vi "Teleop.vi"(10 "Match Info":T1={"Autonomous Elapsed Seconds"=0.0, "TeleOp Elapsed Seconds"=0.0, "Disabled Elapsed Seconds"=0.0, "Visited Autonomous"=FALSE, "Visited TeleOp"=FALSE, "Visited Disabled"=FALSE, "Autonomous Settings"={"Autonomous Style"=enum."Independent", "VI Refnum"=refnum}}, 11 "Call Context":T2) -> ()   [LabVIEW 2019]
doc: "This VI is called for each TeleOp packet received from the DS where the robot is not disabled. It is often used to read from the joysticks and update I/O or to update setpoints for timed control loops. It should complete and return within 20 milliseconds or it may miss DS packets."
uses:
  <vilib>/Rock Robotics/WPI/DriverStation/WPI_DriverStationDerivedRobotMode.ctl
  <vilib>/Rock Robotics/WPI/DriverStation/WPI_DriverStationMatch Info.ctl
  <vilib>/Rock Robotics/WPI/Solenoid/WPI_SolenoidValue.ctl
  <vilib>/Rock Robotics/Network Tables/NT Read Boolean.vi
  <vilib>/Rock Robotics/Network Tables/NT Read Number.vi
  <vilib>/Rock Robotics/WPI/Utilities/WPI_GetSetVariantRefNum.vi
  <vilib>/Rock Robotics/Network Tables/NT Write Boolean Array.vi
  <vilib>/Rock Robotics/Network Tables/NT Write Numeric Array.vi
  <vilib>/Rock Robotics/WPI/RobotDrive/WPI_RobotDriveArcadeDrive_Standard(NoSaturation).vi
  <vilib>/Rock Robotics/WPI/Solenoid/WPI_SolenoidSetEnum.vi
panel:
  out "Sample Slider 0":dbl(slide) scale=0.0..5.0
  out "Sample Boolean 1":bool
  out "Sample Boolean 0":bool
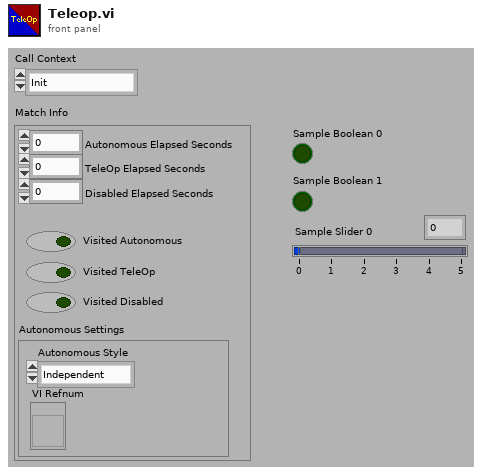
[diagram p1: front panel]
types:
  T1 = typedef "WPI_DriverStationMatch Info.ctl" = cluster{"Autonomous Elapsed Seconds":dbl, "TeleOp Elapsed Seconds":dbl, "Disabled Elapsed Seconds":dbl, "Visited Autonomous":bool, "Visited TeleOp":bool, "Visited Disabled":bool, "Autonomous Settings":cluster{"Autonomous Style":enum16{"Iterative", "Independent"}, "VI Refnum":refnum<vi>}}
  T2 = typedef "WPI_DriverStationDerivedRobotMode.ctl" = enum16{"Init", "Execute", "Stop"}
  T3 = typedef "WPI_JoystickDevRef.ctl" = cluster{"Device":T4}
  T4 = typedef "WPI_JoystickDeviceEnum.ctl" = enum16{"USB 0", "USB 1", "USB 2", "USB 3", "USB 4", "USB 5"}
  T5 = typedef "WPI_MotorControlDeviceRef.ctl" = cluster{"DeviceStatus":errorcluster, "Type":T6, "PWM":cluster{"PWM Channel":T7, "DeadBand":T8}, "CAN":cluster{"Device Number":u8, "SetOutput VI Ref":variant, "GetOutput VI Ref":variant, "Enable VI Ref":variant, "Disable VI Ref":variant, "Data":variant}, "Invert":bool, "DIO PWM":cluster{"PWM \"Enable\" Channel":T7, "DIOChannel":T9, "PWM Rate":dbl}}
  T6 = typedef "WPI_MotorControlType.ctl" = enum16{"PWM", "CAN", "DIO PWM"}
  T7 = typedef "FPGA_DIOPWMChannel.ctl" = enum8{"PWM 0", "PWM 1", "PWM 2", "PWM 3", "PWM 4", "PWM 5", "PWM 6", "PWM 7", "PWM 8", "PWM 9", "PWM MXP 0", "PWM MXP 1", "PWM MXP 2", "PWM MXP 3", "PWM MXP 4", "PWM MXP 5", "PWM MXP 6", "PWM MXP 7", "PWM MXP 8", "PWM MXP 9", "Invalid"}
  T8 = typedef "WPI_PWMDeadband.ctl" = cluster{"Name":string, "maxPositivePwm":i32, "minPositivePwm":i32, "centerPwm":i32, "maxNegativePwm":i32, "minNegativePwm":i32, "angularRange":u16}
  T9 = typedef "FPGA_DIOChannel.ctl" = enum8{"DIO 0", "DIO 1", "DIO 2", "DIO 3", "DIO 4", "DIO 5", "DIO 6", "DIO 7", "DIO 8", "DIO 9", "DIO MXP 0", "DIO MXP 1", "DIO MXP 2", "DIO MXP 3", "DIO MXP 4", "DIO MXP 5", "DIO MXP 6", "DIO MXP 7", "DIO MXP 8", "DIO MXP 9", "DIO MXP 10", "DIO MXP 11", "DIO MXP 12", "DIO MXP 13", "DIO MXP 14", "DIO MXP 15", "SPI Port CS1", "SPI Port CS2", "SPI Port CS3", "SPI Port MISO", "SPI Port MOSI", "Invalid"}
  T10 = typedef "WPI_SolenoidValue.ctl" = enum16{"Off", "On", "Forward", "Reverse"}
  T11 = typedef "WPI_SolenoidDevRef.ctl" = cluster{"DevStatus":errorcluster, "Pneumatics Control Module":u8, "Forward Solenoid Channel":T12, "Reverse Solenoid Channel":T12}
  T12 = typedef "WPI_SolenoidChannel.ctl" = enum8{"Solenoid 0", "Solenoid 1", "Solenoid 2", "Solenoid 3", "Solenoid 4", "Solenoid 5", "Solenoid 6", "Solenoid 7", "Invalid"}
  T13 = typedef "WPI_RobotDriveDevRef.ctl" = cluster{"DevStatus":errorcluster, "Motors[]":T5[], "Square Inputs":bool, "Max Output":dbl}
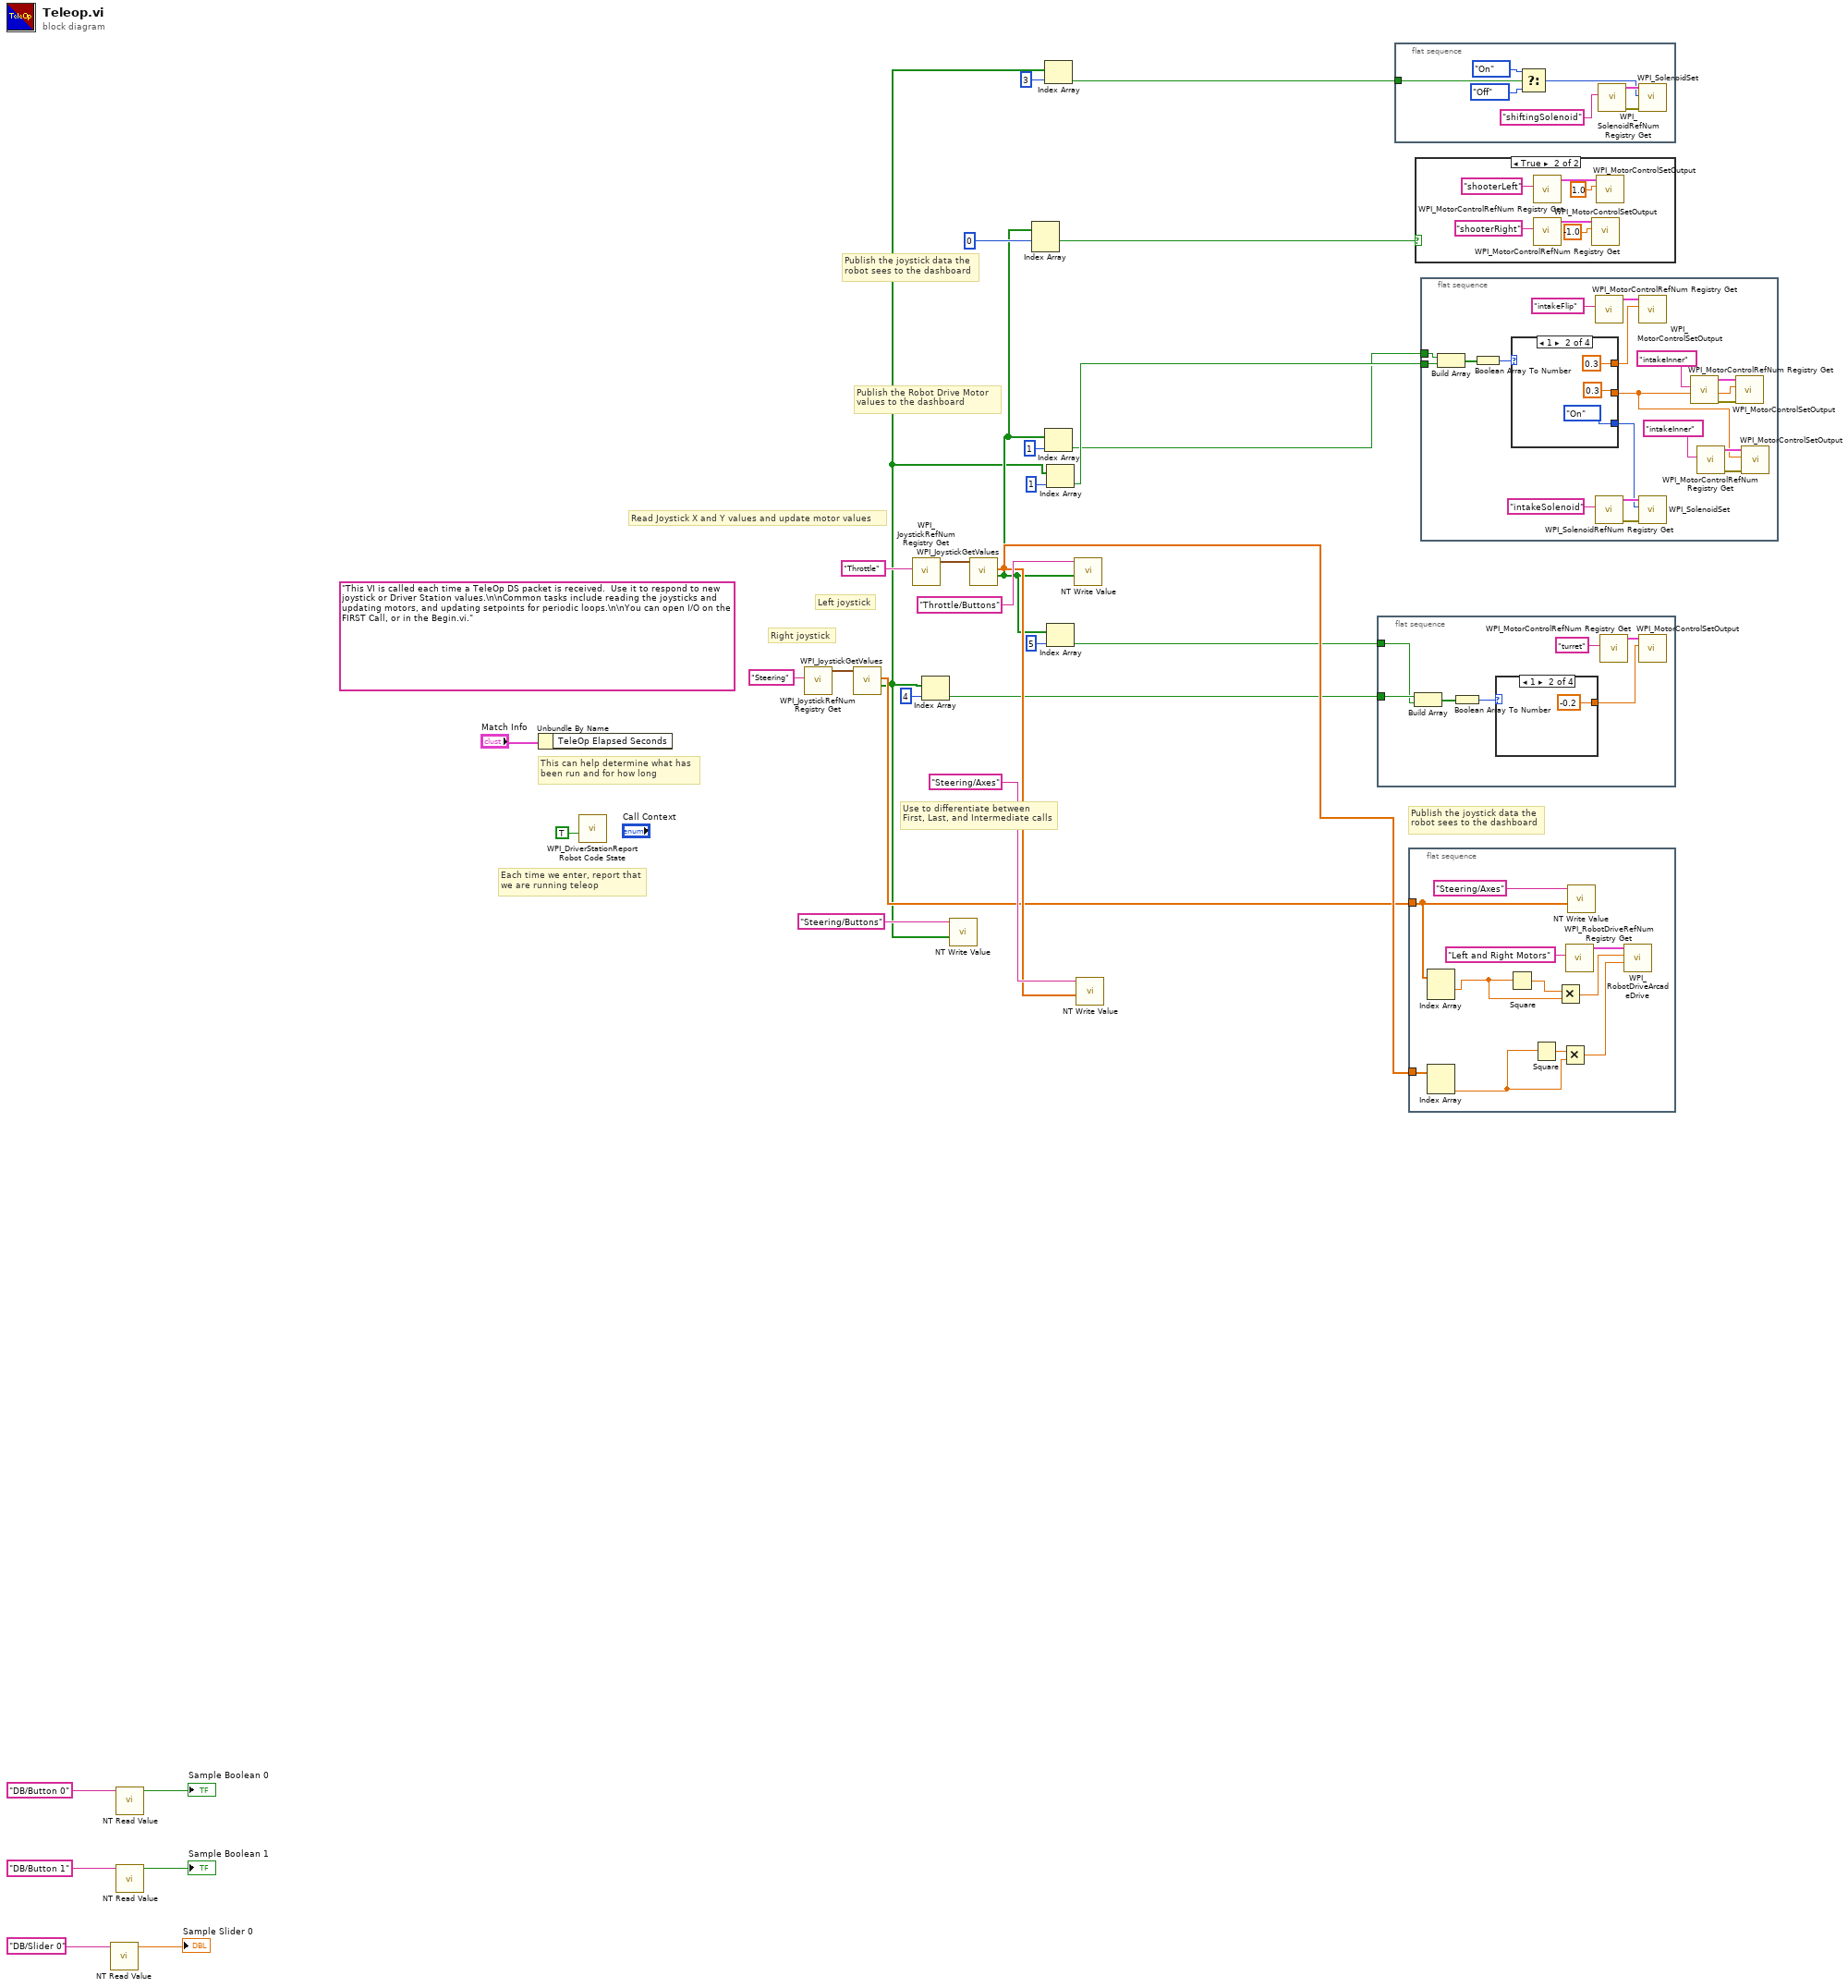
[diagram p0: block diagram]
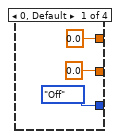
[diagram p2: hidden frame]
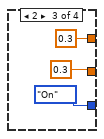
[diagram p3: hidden frame]
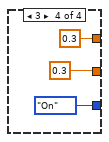
[diagram p4: hidden frame]
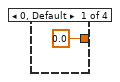
[diagram p5: hidden frame]
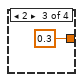
[diagram p6: hidden frame]
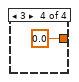
[diagram p7: hidden frame]
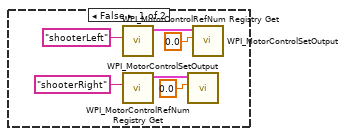
[diagram p8: hidden frame]
diagram:
  (unwired) "This VI is called each time a TeleOp DS packet is received.  Use it to respond to new joystick or Driver Station values.\n\nCommon tasks include reading the joysticks and updating motors, and updating setpoints for periodic loops.\n\nYou can open I/O on the FIRST Call, or in the Begin.vi."
  # "Right joystick"
  # "Left joystick"
  # "Publish the Robot Drive Motor\nvalues to the dashboard"
  # "Publish the joystick data the\nrobot sees to the dashboard"
  # "Publish the joystick data the\nrobot sees to the dashboard"
  # "Each time we enter, report that\nwe are running teleop"
  # "Use to differentiate between\nFirst, Last, and Intermediate calls"
  # "This can help determine what has\nbeen run and for how long"
  # "Read Joystick X and Y values and update motor values"
  n1 = call-poly <vilib>:"NT Read Value.vi"("Name"="DB/Slider 0" ("refnum name")) -> ("Numeric"=→"Sample Slider 0":dbl)  [unwired: 9 in, 1 out]
  n2 = call-poly <vilib>:"NT Read Value.vi"("Name"="DB/Button 0" ("refnum name")) -> ("Boolean"=→"Sample Boolean 0":bool)  [unwired: 9 in, 1 out]
  n3 = call-poly <vilib>:"NT Read Value.vi"("Name"="DB/Button 1" ("refnum name")) -> ("Boolean"=→"Sample Boolean 1":bool)  [unwired: 9 in, 1 out]
  n4 = Unbundle By Name("Match Info") -> ()  [unwired: 1 out]
  n5 = call <vilib>:"WPI_DriverStationReport Robot Code State.vi"("TeleOp"=TRUE ("Autonomous")) -> ()  [unwired: 10 in, 1 out]
  n6 = call <vilib>:"WPI_JoystickRefNum Registry Get.vi"("refnum name"="Steering") -> ("JoystickDevRef"=w16:T3)  [unwired: 1 in, 9 out]
  n7 = call <vilib>:"WPI_JoystickGetValues.vi"("JoystickDevRef"=w16) -> ("Buttons"=w1:bool[], "Axes"=w14:dbl[])  [unwired: 6 in, 3 out]
  n8 = call <vilib>:"WPI_JoystickRefNum Registry Get.vi"("refnum name"="Throttle") -> ("JoystickDevRef"=w22:T3)  [unwired: 1 in, 9 out]
  n9 = Index Array(array=w1, index=4) -> (element=w9:bool)
  n10 = call-poly <vilib>:"NT Write Value.vi"("Boolean Array"=w1, "Name"="Steering/Buttons") -> ()  [unwired: 9 in, 1 out]
  n11 = call <vilib>:"WPI_JoystickGetValues.vi"("JoystickDevRef"=w22) -> ("Buttons"=w2:bool[], "Axes"=w19:dbl[])  [unwired: 6 in, 3 out]
  n12 = Index Array(array=w2, index #1=0 ("index")) -> (element #1=w7:bool)  [unwired: 1 in, 1 out]
  n13 = Index Array(array=w1, index=3) -> (element=w11:bool)
  n14 = Index Array(array=w2, index=1) -> (element=w3:bool)
  n15 = Index Array(array=w1, index=1) -> (element=w5:bool)
  n16 = Index Array(array=w2, index=5) -> (element=w10:bool)
  n17 = call-poly <vilib>:"NT Write Value.vi"("Boolean Array"=w2, "Name"="Throttle/Buttons") -> ()  [unwired: 9 in, 1 out]
  n18 = call-poly <vilib>:"NT Write Value.vi"("Numeric Array"=w19, "Name"="Steering/Axes") -> ()  [unwired: 9 in, 1 out]
  n19 = flat-sequence {
    tunnel: w9 -> [w38]
    tunnel: w10 -> [w37]
    frame #0 {
      n20 = Build Array(w38, w37) -> (w36:bool[])
      n21 = Boolean Array To Number(Boolean array=w36) -> (number=w35:u32)
      n22 = case shown="1" w35 {
        tunnel: [0.0 ("f") -0.2 ("f") 0.3 ("f") 0.0 ("f")] -> w32
        frame 0, Default {
        }
        frame 1 {
        }
        frame 2 {
        }
        frame 3 {
        }
      }
      n23 = call <vilib>:"WPI_MotorControlRefNum Registry Get.vi"("refnum name"="turret") -> ("MotorControlDevRef"=w34:T5)  [unwired: 9 in, 1 out]
      n24 = call <vilib>:"WPI_MotorControlSetOutput.vi"("Output"=w32, "MotorControlDevRef"=w34) -> ()  [unwired: 7 in, 3 out]
    }
  }
  n25 = flat-sequence {
    tunnel: w11 -> [w46]
    frame #0 {
      n26 = Select(t=WPI_SolenoidValue."On" ("Value"), s=w46, f=WPI_SolenoidValue."Off" ("Value")) -> (s? t:f=w43:T10)
      n27 = call <vilib>:"WPI_SolenoidRefNum Registry Get.vi"("refnum name"="shiftingSolenoid") -> ("error out"=w47:errorcluster, "SolenoidDevRef"=w49:T11)  [unwired: 9 in]
      n28 = call-poly <vilib>:"WPI_SolenoidSet.vi"("error in (no error)"=w47, "Value"=w43, "SolenoidDevRef"=w49) -> ()  [unwired: 7 in, 2 out]
    }
  }
  n29 = flat-sequence {
    tunnel: w19 -> [w59]
    tunnel: w14 -> [w56]
    frame #0 {
      n30 = Index Array(array=w56) -> (element #1=w54:dbl)  [unwired: 2 in, 1 out]
      n31 = Index Array(array=w59) -> (element #2=w52:dbl)  [unwired: 2 in, 1 out]
      n32 = Square(x=w54) -> (x^2=w55:dbl)
      n33 = Square(x=w52) -> (x^2=w51:dbl)
      n34 = Multiply(x=w55, y=w54) -> (x*y=w53:dbl)
      n35 = Multiply(x=w51, y=w52) -> (x*y=w50:dbl)
      n36 = call <vilib>:"WPI_RobotDriveRefNum Registry Get.vi"("refnum name"="Left and Right Motors") -> ("RobotDriveDevRef"=w58:T13)  [unwired: 1 in, 9 out]
      n37 = call-poly <vilib>:"NT Write Value.vi"("Numeric Array"=w56, "Name"="Steering/Axes") -> ()  [unwired: 9 in, 1 out]
      n38 = call-poly <vilib>:"WPI_RobotDriveArcadeDrive.vi"("Y axis value"=w50, "X axis value"=w53, "RobotDriveDevRef"=w58) -> ()  [unwired: 6 in, 3 out]
    }
  }
  n39 = case shown="True" w7 {
    frame False {
      n40 = call <vilib>:"WPI_MotorControlRefNum Registry Get.vi"("refnum name"="shooterLeft") -> ("MotorControlDevRef"=w66:T5)  [unwired: 9 in, 1 out]
      n41 = call <vilib>:"WPI_MotorControlRefNum Registry Get.vi"("refnum name"="shooterRight") -> ("MotorControlDevRef"=w63:T5)  [unwired: 9 in, 1 out]
      n42 = call <vilib>:"WPI_MotorControlSetOutput.vi"("Output"=0.0, "MotorControlDevRef"=w63) -> ()  [unwired: 7 in, 3 out]
      n43 = call <vilib>:"WPI_MotorControlSetOutput.vi"("Output"=0.0, "MotorControlDevRef"=w66) -> ()  [unwired: 7 in, 3 out]
    }
    frame True {
      n44 = call <vilib>:"WPI_MotorControlRefNum Registry Get.vi"("refnum name"="shooterLeft") -> ("MotorControlDevRef"=w72:T5)  [unwired: 9 in, 1 out]
      n45 = call <vilib>:"WPI_MotorControlRefNum Registry Get.vi"("refnum name"="shooterRight") -> ("MotorControlDevRef"=w69:T5)  [unwired: 9 in, 1 out]
      n46 = call <vilib>:"WPI_MotorControlSetOutput.vi"("Output"=-1.0, "MotorControlDevRef"=w69) -> ()  [unwired: 7 in, 3 out]
      n47 = call <vilib>:"WPI_MotorControlSetOutput.vi"("Output"=1.0, "MotorControlDevRef"=w72) -> ()  [unwired: 7 in, 3 out]
    }
  }
  n48 = flat-sequence {
    tunnel: w3 -> [w90]
    tunnel: w5 -> [w89]
    frame #0 {
      n49 = Build Array(w90, w89) -> (w88:bool[])
      n50 = Boolean Array To Number(Boolean array=w88) -> (number=w87:u32)
      n51 = case shown="1" w87 {
        tunnel: [0.0 ("f") 0.3 ("f") 0.3 ("f") 0.3 ("f")] -> w84
        tunnel: [WPI_SolenoidValue."Off" ("Value") WPI_SolenoidValue."On" ("Value") WPI_SolenoidValue."On" ("Value") WPI_SolenoidValue."On" ("Value")] -> w80
        tunnel: [0.0 ("f") 0.3 ("f") 0.3 ("f") 0.3 ("Output")] -> w73
        frame 0, Default {
        }
        frame 1 {
        }
        frame 2 {
        }
        frame 3 {
        }
      }
      n52 = call <vilib>:"WPI_MotorControlRefNum Registry Get.vi"("refnum name"="intakeFlip") -> ("MotorControlDevRef"=w86:T5)  [unwired: 9 in, 1 out]
      n53 = call <vilib>:"WPI_SolenoidRefNum Registry Get.vi"("refnum name"="intakeSolenoid") -> ("error out"=w81:errorcluster, "SolenoidDevRef"=w83:T11)  [unwired: 9 in]
      n54 = call <vilib>:"WPI_MotorControlSetOutput.vi"("Output"=w84, "MotorControlDevRef"=w86) -> ()  [unwired: 7 in, 3 out]
      n55 = call-poly <vilib>:"WPI_SolenoidSet.vi"("error in (no error)"=w81, "Value"=w80, "SolenoidDevRef"=w83) -> ()  [unwired: 7 in, 2 out]
      n56 = call <vilib>:"WPI_MotorControlRefNum Registry Get.vi"("refnum name"="intakeInner") -> ("error out"=w77:errorcluster, "MotorControlDevRef"=w78:T5)  [unwired: 9 in]
      n57 = call <vilib>:"WPI_MotorControlRefNum Registry Get.vi"("refnum name"="intakeInner") -> ("error out"=w74:errorcluster, "MotorControlDevRef"=w75:T5)  [unwired: 9 in]
      n58 = call <vilib>:"WPI_MotorControlSetOutput.vi"("error in (no error)"=w77, "Output"=w73, "MotorControlDevRef"=w78) -> ()  [unwired: 6 in, 3 out]
      n59 = call <vilib>:"WPI_MotorControlSetOutput.vi"("error in (no error)"=w74, "Output"=w73, "MotorControlDevRef"=w75) -> ()  [unwired: 6 in, 3 out]
    }
  }
